vi "Get SMO HELP.vi"(8 "error in (no error)":errorcluster, 10 "Command":string, 11 "Instrument.Strain in":refnum<class "Instrument.Strain.lvclass">) -> (0 "error out":errorcluster, 2 "help cluster":T1, 3 "Instrument.Strain out":refnum<class "Instrument.Strain.lvclass">)   [LabVIEW 2019, in "Instrument.Strain.lvclass"]
uses:
  Instrument.Strain.lvclass
  Instrument/Help/typedefs/Help--cluster.ctl
  Typedefs/Strain.Commands--Enum.ctl
  Typedefs/setStrain--cluster.ctl
  Instrument/Instrument.lvclass
  Instrument/Help/Help.lvclass
  Instrument/Typedefs/Instrument.Commands--Enum.ctl
  Instrument/Typedefs/Instrument.IDN--cluster.ctl
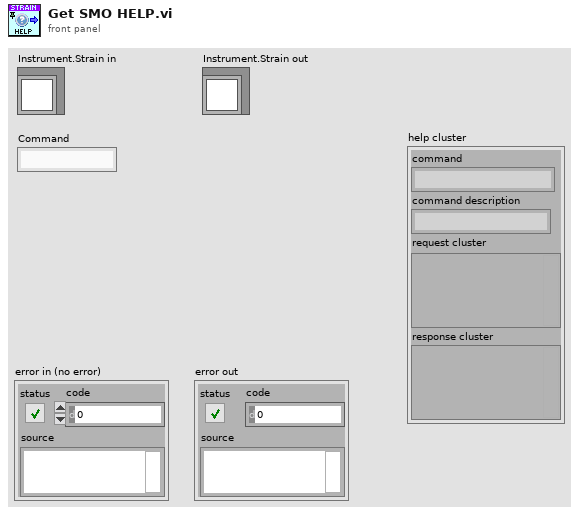
[diagram p1: front panel]
types:
  T1 = typedef "Help.lvclass/Help--cluster.ctl" = cluster{"command":string, "command description":string, "request cluster":variant, "response cluster":variant}
  T2 = typedef "Instrument.Strain.lvclass/setStrain--cluster.ctl" = cluster{"strain":dbl, "slew":dbl, "channel":i32}
  T3 = typedef "Instrument.lvclass/Instrument.Commands--Enum.ctl" = enum16{"ACK", "HELP", "IDN", "getAll", "getAllData"}
  T4 = typedef "Instrument.lvclass/Instrument.IDN--cluster.ctl" = cluster{"vendor":string, "model":string, "serial":string, "firmware":string}
  T5 = typedef "Instrument.Strain.lvclass/Strain.Commands--Enum.ctl" = enum16{"getStrain", "setStrain"}
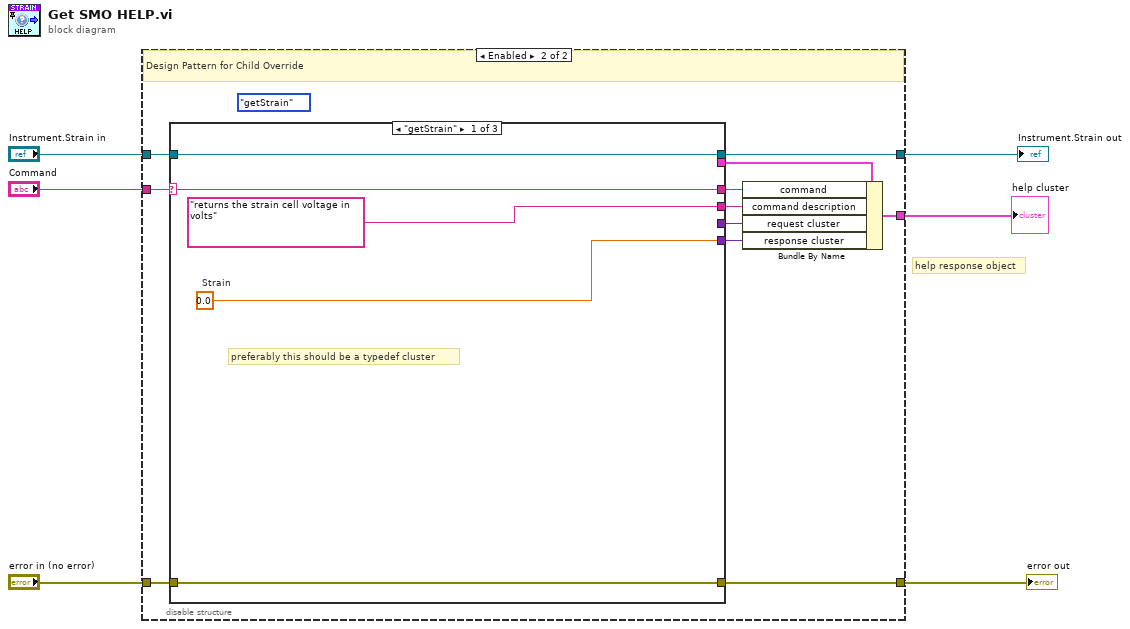
[diagram p0: block diagram]
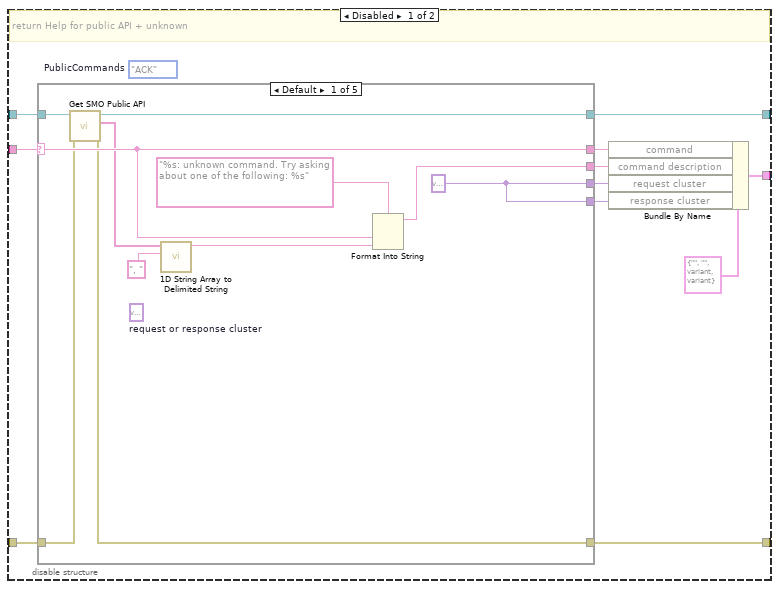
[diagram p2: hidden frame]
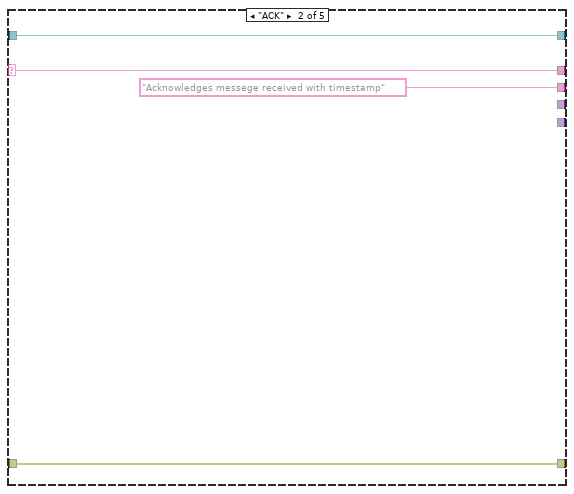
[diagram p3: hidden frame]
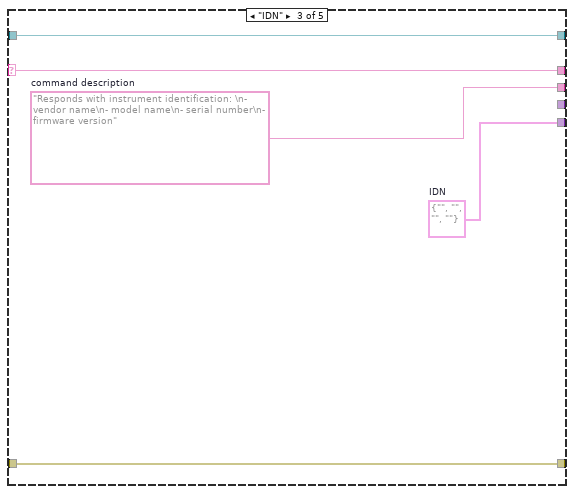
[diagram p4: hidden frame]
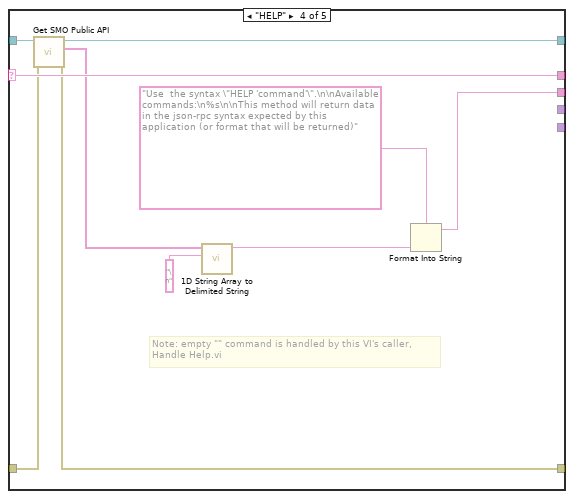
[diagram p5: hidden frame]
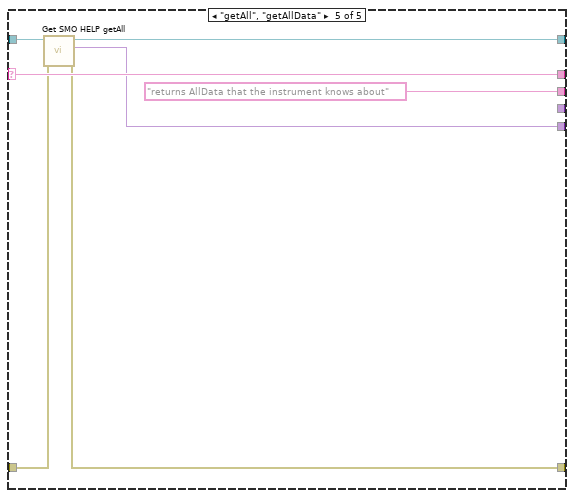
[diagram p6: hidden frame]
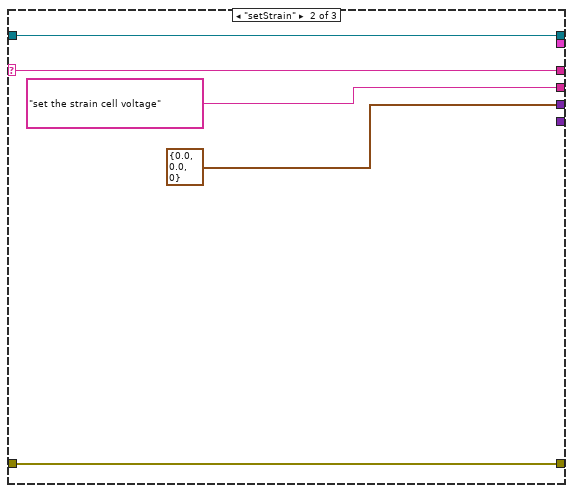
[diagram p7: hidden frame]
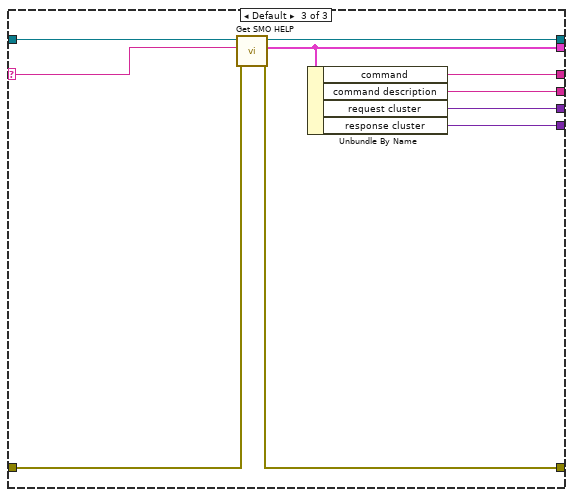
[diagram p8: hidden frame]
diagram:
  # "help response object"
  n1 = disable-structure shown="Enabled" {
    disable-tunnel: [w17 w56] -> w4
    disable-tunnel: "Instrument.Strain in" -> [w16 w57]
    disable-tunnel: "error in (no error)" -> [w15 w63]
    disable-tunnel: [w11 w65] -> w6
    disable-tunnel: [w8 w64] -> w5
    disable-tunnel: "Command" -> [w7 w62]
    frame Disabled {
      (unwired) Instrument.Commands--Enum."ACK"  # PublicCommands
      # "return Help for public API + unknown"
      n2 = case shown="Default" w7 {
        selector: w7 -> [w24 w30 w36 w44 w53]
        tunnel: w15 -> [w21 w32 w33 w40 w52]
        tunnel: [w22 w32 w33 w41 w51] -> w11
        tunnel: [w26 "Acknowledges messege received with timestamp" w37 w43 "returns AllData that the instrument knows about"] -> w13
        tunnel: [w19 _ _ _ _] -> w12
        tunnel: [w19 _ w34 _ w48] -> w10
        tunnel: [w24 w30 w36 w44 w53] -> w14
        tunnel: w16 -> [w23 w29 w35 w42 w49]
        tunnel: [w20 w29 w35 w39 w50] -> w17
        frame Default {
          (unwired) variant  # request or response cluster
          w19 = variant ("response cluster")
          n3 = call-dynamic "Get SMO Public API.vi"("error in (no error)"=w21, "Instrument.Strain in"=w23) -> ("error out"=w22:errorcluster, "commands"=w18:string[], "Instrument.Strain out"=w20:refnum<class "Instrument.Strain.lvclass">)  [unwired: 7 in]
          n4 = call <vilib>:"1D String Array to Delimited String.vi"("delimiter"=", ", "string array"=w18) -> ("delimited string"=w27:string)  [unwired: 9 in]
          n5 = Format Into String(format string="%s: unknown command. Try asking about one of the following: %s", w24, w27) -> (resulting string=w26:string)  [unwired: 2 in, 1 out]
        }
        frame "ACK" {
        }
        frame "IDN" {
          w34 = T4 {"vendor"="", "model"="", "serial"="", "firmware"=""}  # IDN
          w37 = "Responds with instrument identification: \n- vendor name\n- model name\n- serial number\n- firmware version"  # command description
        }
        frame "HELP" {
          # "Note: empty \"\" command is handled by this VI's caller,\nHandle Help.vi"
          n6 = call-dynamic "Get SMO Public API.vi"("error in (no error)"=w40, "Instrument.Strain in"=w42) -> ("error out"=w41:errorcluster, "commands"=w38:string[], "Instrument.Strain out"=w39:refnum<class "Instrument.Strain.lvclass">)  [unwired: 7 in]
          n7 = call <vilib>:"1D String Array to Delimited String.vi"("delimiter"="\n", "string array"=w38) -> ("delimited string"=w47:string)  [unwired: 9 in]
          n8 = Format Into String(format string="Use  the syntax \"HELP 'command'\".\n\nAvailable commands:\n%s\n\nThis method will return data in the json-rpc syntax expected by this application (or format that will be returned)", w47) -> (resulting string=w43:string)  [unwired: 2 in, 1 out]
        }
        frame "getAll", "getAllData" {
          n9 = call-dynamic "Get SMO HELP getAll.vi"("error in (no error)"=w52, "Instrument in"=w49) -> ("error out"=w51:errorcluster, "response cluster"=w48:variant, "Instrument out"=w50:refnum<class "Instrument.Strain.lvclass">)  [unwired: 7 in]
        }
      }
      n10 = Bundle By Name(cluster=T1 {"command"="", "command description"="", "request cluster"=variant, "response cluster"=variant} ("Help"), "command"=w14, "command description"=w13, "request cluster"=w12, "response cluster"=w10) -> (w8:T1)
    }
    frame Enabled {
      (unwired) Strain.Commands--Enum."getStrain" ("Command")
      # "Design Pattern for Child Override"
      n11 = case shown="\"getStrain\"" w62 {
        selector: w62 -> [w70 w75 w80]
        tunnel: [w70 w75 w82] -> w61
        tunnel: w63 -> [w69 w74 w78]
        tunnel: [w69 w74 w77] -> w65
        tunnel: ["returns the strain cell voltage in volts" "set the strain cell voltage" w83] -> w60
        tunnel: [_ T2 {"strain"=0.0, "slew"=0.0, "channel"=0} ("setStrain") w84] -> w59
        tunnel: [w66 _ w85] -> w58
        tunnel: w57 -> [w67 w72 w81]
        tunnel: [w67 w72 w76] -> w56
        tunnel: [_ _ w79] -> w55
        frame "getStrain" {
          w66 = 0.0  # Strain
          # "preferably this should be a typedef cluster"
        }
        frame "setStrain" {
        }
        frame Default {
          n12 = call-parent "Get SMO HELP.vi"("error in (no error)"=w78, "Command"=w80, "Instrument in"=w81) -> ("error out"=w77:errorcluster, "help cluster"=w79:T1, "Instrument out"=w76:refnum<class "Instrument.Strain.lvclass">)  [unwired: 6 in]
          n13 = Unbundle By Name(w79) -> ("command"=w82:string, "command description"=w83:string, "request cluster"=w84:variant, "response cluster"=w85:variant)
        }
      }
      n14 = Bundle By Name(cluster=w55, "command"=w61, "command description"=w60, "request cluster"=w59, "response cluster"=w58) -> (w64:T1)
    }
  }
  "Instrument.Strain out" <- w4
  "help cluster" <- w5
  "error out" <- w6
